vi "Set Section.vi"(8 "error in (no error)":errorcluster, 10 "Section":string, 11 "Object Entry in":refnum<class "OD Section.lvclass">) -> (0 "error out":errorcluster, 3 "Object Entry out":refnum<class "OD Section.lvclass">)   [LabVIEW 2024, in "EDS.lvlib" / "OD Section.lvclass"]
uses:
  OD Section.lvclass
  OD Section.lvclass/OD Section.ctl
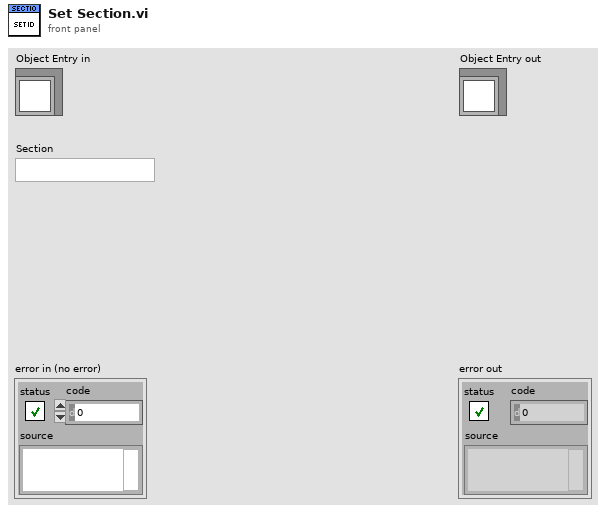
[diagram p1: front panel]
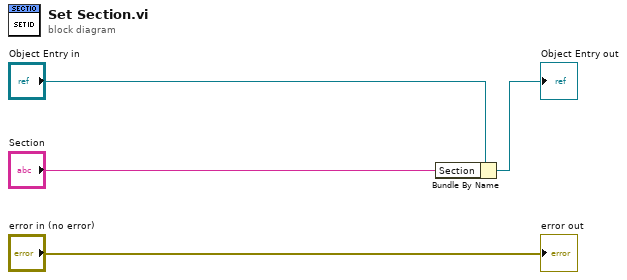
[diagram p0: block diagram]
diagram:
  n1 = Bundle By Name(cluster="Object Entry in", "Section"="Section") -> (→"Object Entry out":refnum<class "OD Section.lvclass">)
  "error out" <- "error in (no error)"
